vi "Write Auto-open.vi"(8 "error in (no error)":errorcluster, 10 "Auto-open":bool, 11 "Mag Lab Measure UI in":refnum<class "Mag Lab Measure UI.lvclass">) -> (0 "error out":errorcluster, 3 "Mag Lab Measure UI out":refnum<class "Mag Lab Measure UI.lvclass">)   [LabVIEW 2015, in "Mag Lab Measure UI.lvclass"]
uses:
  Mag Lab Measure UI.lvclass
  Mag Lab Measure UI.lvclass/Mag Lab Measure UI.ctl
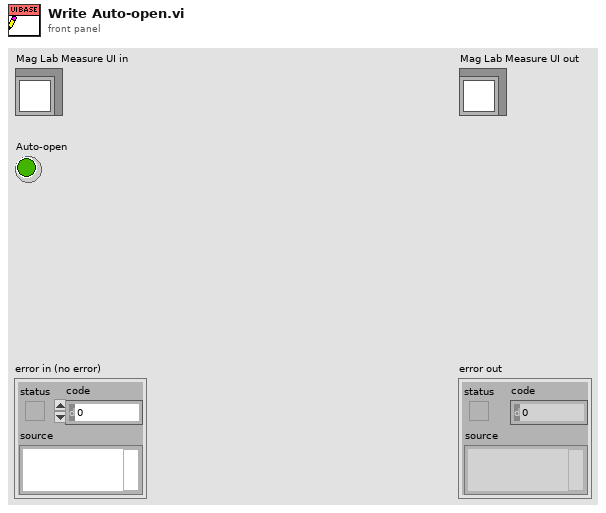
[diagram p1: front panel]
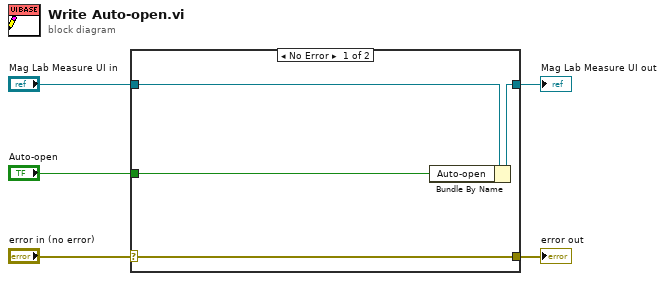
[diagram p0: block diagram]
diagram:
  n1 = case shown="No Error" "error in (no error)" {
    selector: "error in (no error)" -> [w9 w10]
    tunnel: [w9 w10] -> w4
    tunnel: [w7 w11] -> w2
    tunnel: "Mag Lab Measure UI in" -> [w8 w11]
    tunnel: "Auto-open" -> [w6 _]
    frame No Error {
      n2 = Bundle By Name(cluster=w8, "Auto-open"=w6) -> (w7:refnum<class "Mag Lab Measure UI.lvclass">)
    }
    frame Error {
    }
  }
  "error out" <- w4
  "Mag Lab Measure UI out" <- w2
